vi "Add PV (NT).vi"(5 "is read only? (F)":bool, 7 "PV name":string, 8 "error in (no error)":errorcluster, 10 "initial value":refnum<class "NT Base.lvclass">, 11 "Server in":refnum<class "Server.lvclass">) -> (0 "error out":errorcluster, 2 "value out":refnum<class "NT Base.lvclass">, 3 "Server out":refnum<class "Server.lvclass">)   [LabVIEW 2020, in "PV Access.lvlib" / "PVA Server.lvlib" / "Server.lvclass"]
uses:
  Server.lvclass
  PV Data/NT Base/NT Base.lvclass
  Server.lvclass/Server.ctl
  Source/Source.lvclass
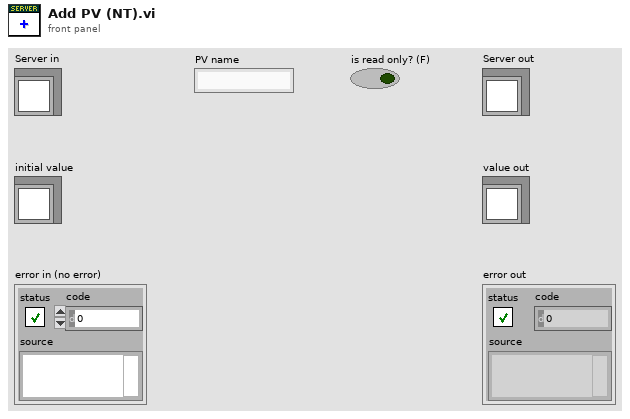
[diagram p1: front panel]
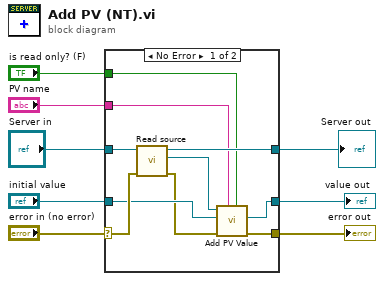
[diagram p0: block diagram]
diagram:
  n1 = case shown="No Error" "error in (no error)" {
    selector: "error in (no error)" -> [w14 w21]
    tunnel: [w13 w21] -> w7
    tunnel: [w17 w20] -> w5
    tunnel: "Server in" -> [w18 w20]
    tunnel: "PV name" -> [w15 _]
    tunnel: "initial value" -> [w12 w19]
    tunnel: [w10 w19] -> w2
    tunnel: "is read only? (F)" -> [w9 _]
    frame No Error {
      n2 = call "Read source.vi"("error in (no error)"=w14, "Server in"=w18) -> ("error out"=w11:errorcluster, "Source"=w16:refnum<class "Source.lvclass">, "Server out"=w17:refnum<class "Server.lvclass">)  [unwired: 7 in]
      n3 = call "Add PV Value.vi"("is read only? (F)"=w9, "PV name"=w15, "error in"=w11, "NT Base in"=w12, "Source in"=w16) -> ("error out"=w13:errorcluster, "NT Base out"=w10:refnum<class "NT Base.lvclass">)  [unwired: 4 in, 1 out]
    }
    frame Error {
    }
  }
  "error out" <- w7
  "Server out" <- w5
  "value out" <- w2
